vi "Send Panel Close.vi"(6 "Name (use VI name)":string, 8 "error in (no error)":errorcluster, 9 "Discarded?":bool, 10 "VI Refnum":refnum<vi>, 11 "Message Enqueuer in":refnum<class "Message Enqueuer.lvclass">) -> (0 "error out":errorcluster)   [LabVIEW 2015, in "ActorAutoRegistration.lvlib" / "PanelCloseMsg.lvclass"]
uses:
  PanelCloseMsg.lvclass
  <vilib>/ActorFramework/Message Enqueuer/Message Enqueuer.lvclass
  PanelCloseMsg.lvclass/PanelCloseMsg.ctl
  EventDataMessage/EventDataMessage.lvclass
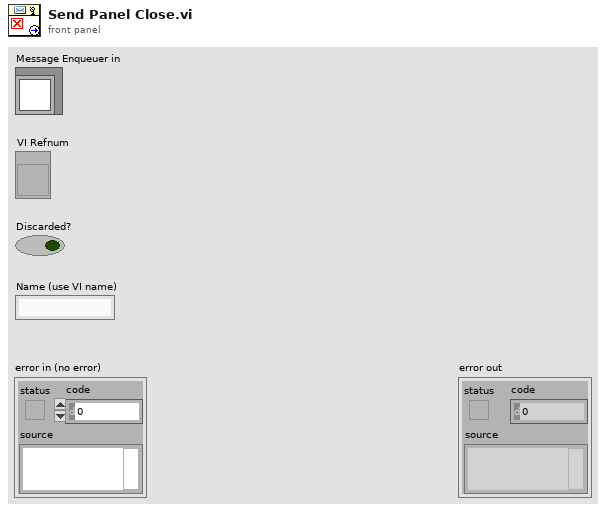
[diagram p1: front panel]
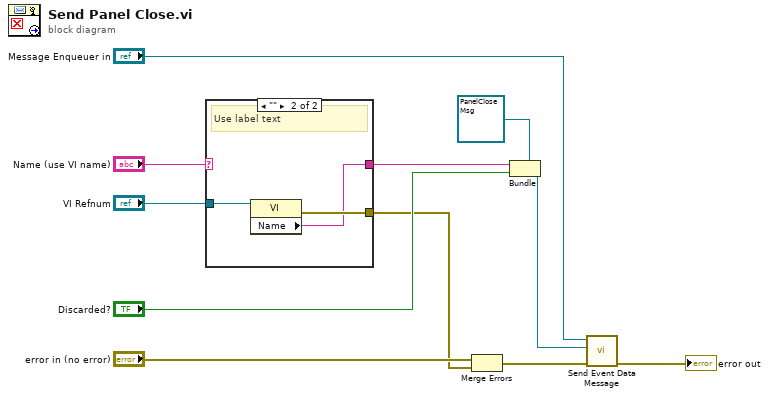
[diagram p0: block diagram]
diagram:
  n1 = case shown="\"\"" "Name (use VI name)" {
    selector: "Name (use VI name)" -> [w12 _]
    tunnel: [w12 w13] -> w11
    tunnel: "VI Refnum" -> [_ w15]
    tunnel: [_ w14] -> w4
    frame Default {
      # "Use string provided"
    }
    frame "" {
      # "Use label text"
      n2 = property class="VI"(reference=w15) -> (error out=w14:errorcluster, "Name"=w13:string)  [unwired: 1 in, 1 out]
    }
  }
  n3 = Merge Errors("error in (no error)", w4) -> (w5:errorcluster)
  n4 = Bundle(cluster=refnum<class "PanelCloseMsg.lvclass"> refnum ("PanelCloseMsg"), w11, "Discarded?") -> (w2:refnum<class "PanelCloseMsg.lvclass">)
  n5 = call "Send Event Data Message.vi"("error in (no error)"=w5, "EventDataMessage in"=w2, "Message Enqueuer in"="Message Enqueuer in") -> ("error out"=→"error out":errorcluster)  [unwired: 8 in]
